vi "Grab images from pco.edge or pco.pixelfly USB with soft ROI.vi"() -> ()   [LabVIEW 2012]
doc: "A short program to demonstrate the fundamentals of control and image acquision with the pco.camera series. The program records a sequence of images, with \"live\" updating, while the \"Record\" button is on. Use ctrl-H for more help on the individual controls and indicators."
panel:
  out "bClose":bool
  in  "Quit":bool
  out "BufNr1":i16
  out "BufNr0":i16
  in  "bUseBuffer1":bool
  in  "bUseBuffer0":bool
  in  "ROIX1":u16=1 min=1
  in  "ROIY1":u16=1 min=1
  in  "ROIY0":u16=1 min=1
  in  "ROIX0":u16=1 min=1
  out "Bits/pixel":u16
  in  "Record":bool
  in  "DelayTimeBase":u16(ring)=2 items=["nanoseconds", "microseconds", "milliseconds"]
  in  "ExposureTimeBase":u16(ring)=2 items=["nanoseconds", "microseconds", "milliseconds"]
  in  "Exposure":u32=10
  in  "Delay":u32
  in  "Rate":i32(ring) items=["12000000", "24000000"]
  out "Image":u16[][](graph)
  in  "TriggerMode":u16(ring) items=["Auto", "Software", "External sequence start ", "External exposure control"]
  # "A short program to demonstrate the fundamentals of control and image acquision with the pco.camera series. The program records a sequence of images, with \"live\" updating, while the \"Record\" button is on.  Use ctrl-H for more help on the individual controls and indicators."
  # "pco.labview"
  # "1) Setup camera:"
  # "2) Record  images:"
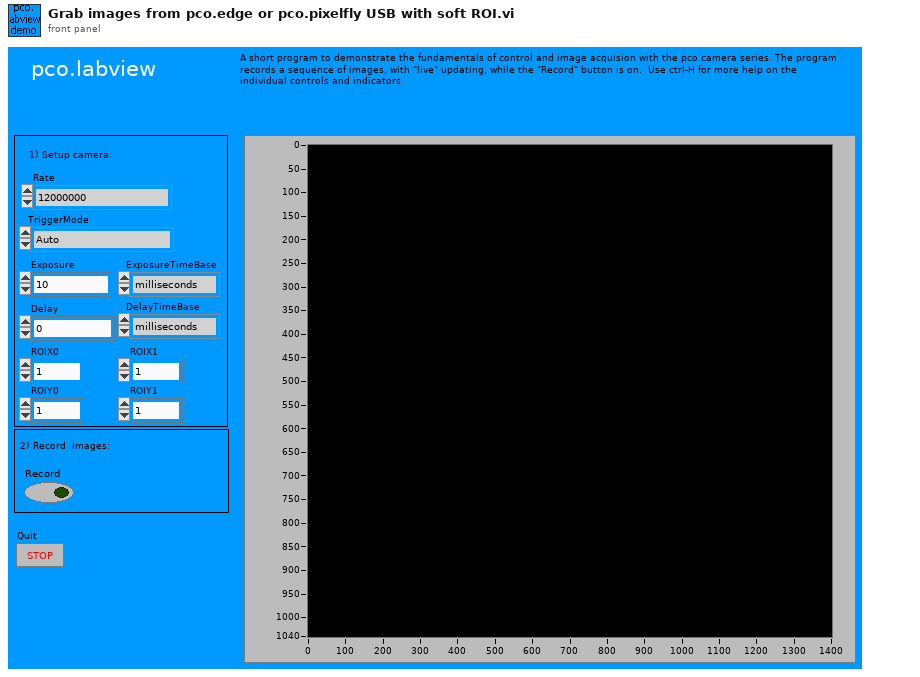
[diagram p1: front panel]
types:
  T1 = cluster{"SSize":u16, "CamType":u16, "CamsSubType":u16, "SerialNumber":u32, "HWVersion":u32, "FWVersion ":u32, "InterfaceType":u16, "HardwareVersions":cluster{"Board":u16, cluster{"string":string, "BatchNumber":u16, "MinorRevision":u8, "MajorRevision":u8, "Variant":u16}[]}, "FirmwareVersions":cluster{"DeviceNum":u16, cluster{"string":string, "MinorRevision":u8, "MajorRevision":u8, "Variant":u16}[]}}
  T2 = cluster{"Size":u16, "SensorTypeDESC":u16, "SensorSubtypeDESC":u16, "MaxHorizontalResStdDESC":u16, "MaxVerticalResStdDESC":u16, "MaxHorizontalResExtDESC":u16, "MaxVerticalResExtDESC":u16, "DynResDESC":u16, "MaxBinHorzDESC":u16, "BinHorzStepDESC":bool, "MaxBinVertDESC":u16, "BinVertStepDESC":bool, "ROIHorzStepDESC":u16, "ROIVertStepDESC":u16, "NumADCDESC":u16, "IRDESC":bool, "MinDelayDESC":u32, "MaxDelayDESC":u32, "MinDelayStepDESC":u32, "MinExpoDESC":u32, "MaxExpoDESC":u32, "MinExpoStepDESC":u32, "MinDelayIRDESC":u32, "MaxDelayIRDESC":u32, "MinExpoIRDESC":u32, "MaxExpoIRDESC":u32, "TimeTableDESC":bool, "DoubleImageDESC":bool, "MinCoolSetDESC":i16, "MaxCoolSetDESC":i16, "MDefaultCoolSetDESC":i16, "PowerDownModeDESC":bool, "OffsetRegDESC":bool, "ColorPattern":cluster{"UpperLeftColor":u8, "UpperRightColor":u8, "LowerLeftColor":u8, "LowerRightColor":u8}, "PatternTypeDESC":bool, "PixelRates":u32[], "CoversionFactors":u16[], "Reserved":u32[], "GeneralCapabilities":u32, "GeneralCapabilities 2":u32, "Min Size Hor":u16, "Min Size Vert":u16, "Ext Synch Freq":u32[], "Cooling Setpoints":i16[], "Soft ROI Hor Step":u16, "Soft ROI Vert Step":u16}
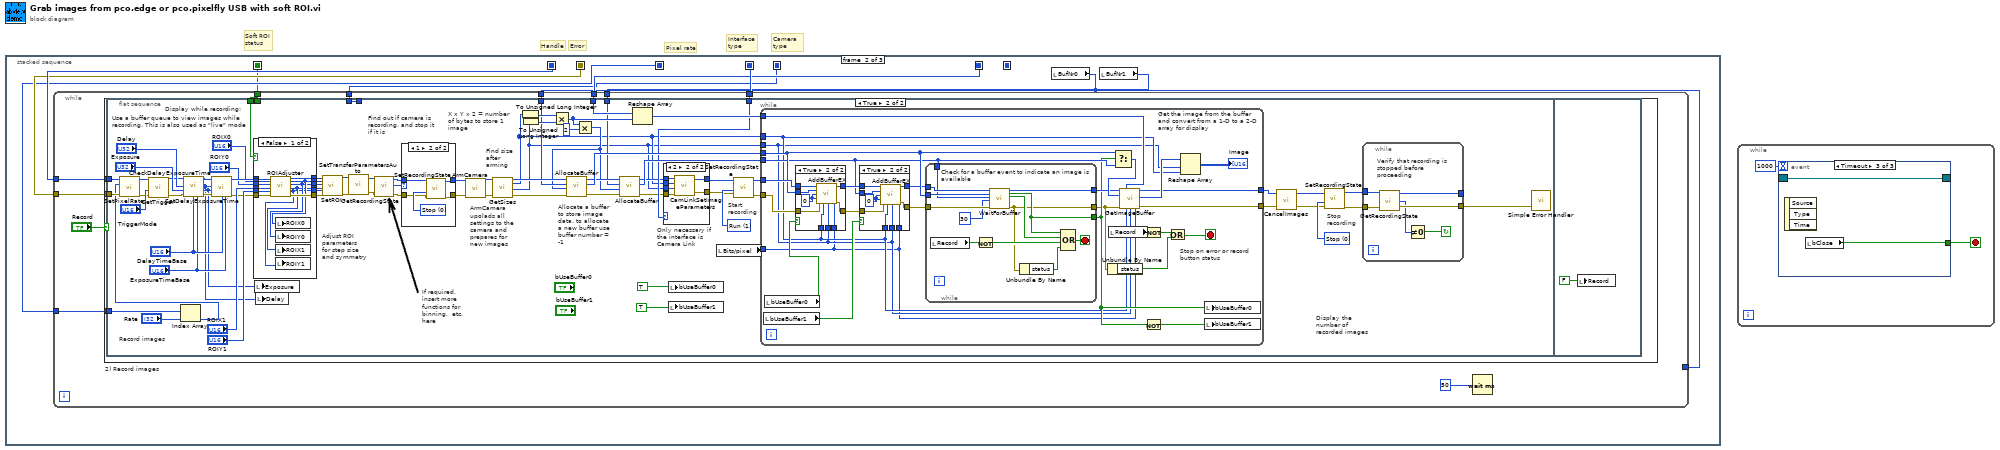
[diagram p0: block diagram]
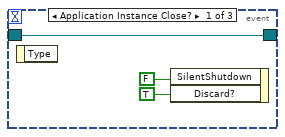
[diagram p2: hidden frame]
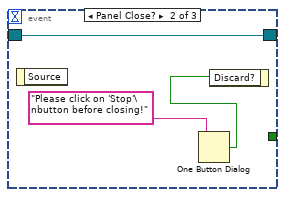
[diagram p3: hidden frame]
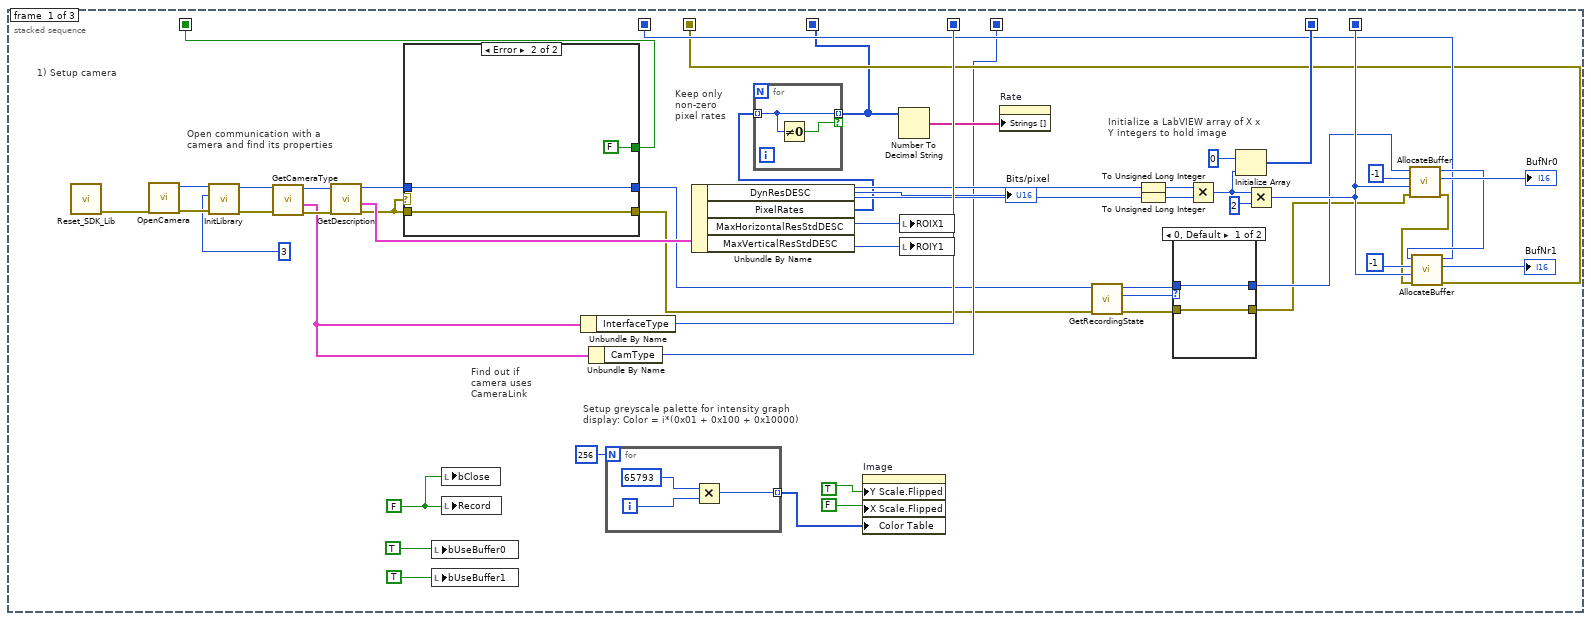
[diagram p4: hidden frame]
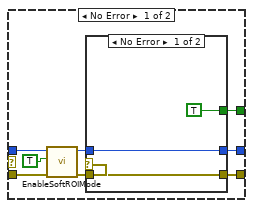
[diagram p5: hidden frame]
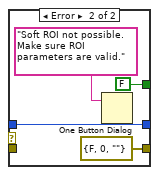
[diagram p6: hidden frame]
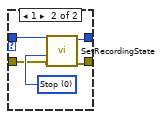
[diagram p7: hidden frame]
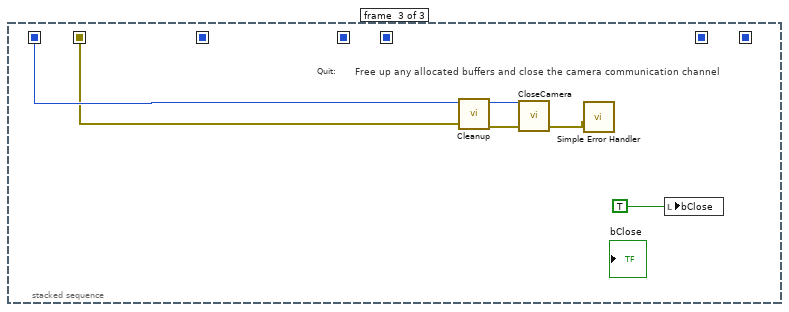
[diagram p14: hidden frame]
diagram:
  # "Soft ROI\nstatus"
  # "Camera type"
  # "Interface type"
  # "Error"
  # "Handle"
  # "Pixel rate"
  n1 = stacked-sequence {
    seq-local: [w44 _ _] -> [_ w86 _]
    seq-local: [w32 _ _] -> [_ _ _]
    seq-local: [w14 _ _] -> [_ w89 w292]
    seq-local: [w13 _ _] -> [_ w88 w291]
    seq-local: [w39 _ _] -> [_ w87 _]
    seq-local: [w1 _ _] -> [_ w83 _]
    seq-local: [w8 _ _] -> [_ w82 _]
    seq-local: [w3 _ _] -> [_ w81 _]
    frame #0 {
      w26 = FALSE ("stop")
      # "Keep only non-zero pixel rates"
      # "1) Setup camera"
      # "Find out if camera uses CameraLink"
      # "Setup greyscale palette for intensity graph display: Color = i*(0x01 + 0x100 + 0x10000)"
      # "Initialize a LabVIEW array of X x Y integers to hold image"
      # "Open communication with a camera and find its properties"
      n2 = call "Reset_SDK_Lib.vi"() -> ("ErrorOut"=w10:errorcluster)  [unwired: 11 in]
      n3 = call "OpenCamera.vi"("ErrorIn"=w10) -> ("ErrorOut"=w23:errorcluster, "Handle out"=w24:u64)  [unwired: 3 in, 2 out]
      n4 = call "InitLibrary.vi"("error in (no error)"=w23, "InterfaceType"=u32 3, "ph"=w24) -> ("error out"=w22:errorcluster, "hout"=w21:u64)  [unwired: 7 in]
      n5 = call "GetCameraType.vi"("ph"=w21, "error in (no error)"=w22) -> ("hout"=w41:u64, "CameraType"=w9:T1, "error out"=w40:errorcluster)  [unwired: 1 in, 1 out]
      n6 = call "GetDescription.vi"("ErrorIn"=w40, "ph"=w41) -> ("ErrorOut"=w4:errorcluster, "Description"=w43:T2, "hout"=w7:u64)  [unwired: 2 in, 1 out]
      n7 = case shown="Error" w4 {
        tunnel: w7 -> [w60 w70]
        tunnel: [w56 w70] -> w6
        tunnel: w4 -> [w58 w69]
        tunnel: [w55 w69] -> w5
        tunnel: [w53 FALSE] -> w3
        frame No Error {
          n8 = call "EnableSoftROIMode.vi"("error in (no error)"=w58, "SoftROI"=TRUE, "ph"=w60) -> ("error out"=w54:errorcluster, "hout"=w57:u64)  [unwired: 3 in, 1 out]
          n9 = case shown="No Error" w54 {
            tunnel: w57 -> [w63 w67]
            tunnel: [w63 w67] -> w56
            tunnel: w54 -> [w62 _]
            tunnel: [w62 errorcluster {"status"=FALSE, "code"=0, "source"=""} ("error out")] -> w55
            tunnel: [TRUE FALSE] -> w53
            frame No Error {
            }
            frame Error {
              n10 = One Button Dialog(message="Soft ROI not possible. Make sure ROI parameters are valid.") -> ()  [unwired: 1 in, 1 out]
            }
          }
        }
        frame Error {
        }
      }
      n11 = local write "bUseBuffer0"(TRUE) -> ()
      n12 = local write "bUseBuffer1"(TRUE) -> ()
      n13 = local write "bClose"(w26) -> ()
      n14 = local write "Record"(w26) -> ()
      n15 = Unbundle By Name(w9) -> ("InterfaceType"=w39:u16)
      n16 = Unbundle By Name(w9) -> ("CamType"=w8:u16)
      n17 = for {
        N: 256 -> [_]
        tunnel: [w78] -> w47 mode=indexing
        i -> [w79]
        n18 = Multiply(x=65793, y=w79) -> (x*y=w78:i32)
      }
      n19 = Unbundle By Name(w43) -> ("DynResDESC"=→"Bits/pixel":u16, "PixelRates"=w2:u32[], "MaxHorizontalResStdDESC"=w37:u16, "MaxVerticalResStdDESC"=w36:u16)
      n20 = for {
        tunnel: w2 -> [w52] mode=indexing
        tunnel: [w52] -> w1 mode=indexing if=w51
        n21 = Not Equal To 0?(x=w52) -> (x != 0?=w51:bool)
      }
      n22 = property on="Image" class="IntGraph (strict)"("Y Scale.Flipped"=TRUE, "X Scale.Flipped"=FALSE, "Color Table"=w47) -> ()  [unwired: 2 in, 2 out]
      n23 = Number To Decimal String(number=w1) -> (decimal integer string=w25:string[])  [unwired: 1 in]
      n24 = local write "ROIX1"(w37) -> ()
      n25 = local write "ROIY1"(w36) -> ()
      n26 = property on="Rate" class="Ring (strict)"("Strings []"=w25) -> ()  [unwired: 2 in, 2 out]
      n27 = call "GetRecordingState.vi"("ErrorIn"=w5, "ph"=w6) -> ("ErrorOut"=w17:errorcluster, "Error"=w11:i32, "hout"=w18:u64)  [unwired: 2 in, 1 out]
      n28 = To Unsigned Long Integer(number=w37) -> (unsigned 32bit integer=w34:u32)
      n29 = To Unsigned Long Integer(number=w36) -> (unsigned 32bit integer=w33:u32)
      n30 = case shown="0, Default" w11 {
        tunnel: w18 -> [w72 w76]
        tunnel: w17 -> [w71 w75]
        tunnel: [w72 w74] -> w16
        tunnel: [w71 w73] -> w12
        frame 0, Default {
        }
        frame 1 {
          w77 = u16 0 items=["Stop", "Run"] ("RecordingState")
          n31 = call "SetRecordingState.vi"("ErrorIn"=w75, "RecordingState"=w77, "ph"=w76) -> ("ErrorOut"=w73:errorcluster, "hout"=w74:u64)  [unwired: 2 in, 1 out]
        }
      }
      n32 = Multiply(x=w34, y=w33) -> (x*y=w45:u32)
      n33 = Initialize Array(u16 0 ("Element Data"), w45) -> (w44:u16[])
      n34 = Multiply(x=w45, y=u32 2) -> (x*y=w32:u32)
      n35 = call "AllocateBuffer.vi"("error in (no error)"=w12, "Size"=w32, "BufNr"=i16 -1, "ph"=w16) -> ("error out"=w19:errorcluster, "BufNrOut"=→"BufNr0":i16, "hout"=w15:u64)  [unwired: 2 in, 3 out]
      n36 = call "AllocateBuffer.vi"("error in (no error)"=w19, "Size"=w32, "BufNr"=i16 -1, "ph"=w15) -> ("error out"=w13:errorcluster, "BufNrOut"=→"BufNr1":i16, "hout"=w14:u64)  [unwired: 2 in, 3 out]
    }
    frame #1 {
      n37 = local read "BufNr0"() -> (w85:i16)
      n38 = local read "BufNr1"() -> (w84:i16)
      n39 = while {
        tunnel: w85 -> [_]
        tunnel: w85 -> [w96]
        tunnel: w86 -> [w98]
        tunnel: w87 -> [w99]
        tunnel: w88 -> [w97]
        tunnel: w89 -> [w94]
        tunnel: w84 -> [w95]
        tunnel: w83 -> [w92]
        tunnel: w82 -> [w91]
        tunnel: w81 -> [w90]
        stop <- "Quit" stop-if-true
        n40 = case "2) Record images" shown="True" "Record" {
          tunnel: w94 -> [_ w110]
          tunnel: w97 -> [_ w109]
          tunnel: w99 -> [_ w103]
          tunnel: w98 -> [_ w108]
          tunnel: w96 -> [_ w107]
          tunnel: w95 -> [_ w106]
          tunnel: w92 -> [_ w105]
          tunnel: w91 -> [_ w104]
          tunnel: w90 -> [_ w102]
          frame False {
          }
          frame True {
            n41 = flat-sequence {
              tunnel: w110 -> [w174]
              tunnel: w109 -> [w173]
              tunnel: w108 -> [w170]
              tunnel: w107 -> [w163]
              tunnel: w106 -> [w159]
              tunnel: w105 -> [w146]
              tunnel: w104 -> [_]
              tunnel: w103 -> [w140]
              tunnel: w102 -> [w121]
              frame #0 {
                w185 = u16 1 items=["Stop", "Run"] ("RecordingState")
                w188 = u16 0 items=["Stop", "Run"] ("RecordingState")
                # "Adjust ROI parameters   for step size and symmetry"
                # "Only necessary if the interface is Camera Link"
                # "Display the number of recorded images"
                # "Record images"
                # "Start recording"
                # "Allocate a buffer to store image data. to allocate a new buffer use buffer number = -1"
                # "Find size after arming"
                # "ArmCamera upolads all settings to the camera and prepares for new images"
                # "Find out if camera is recording, and stop it if it is"
                # "If required, insert more functions for binning.  etc. here"
                # "X x Y x 2 = number of bytes to store 1 image"
                # "Stop recording"
                # "Use a buffer queue to view images while recording. This is also used as \"live\" mode"
                # "Display while recording:"
                n42 = Index Array(array=w146, index="Rate") -> (element=w145:u32)
                n43 = call "SetPixelRate.vi"("error in (no error)"=w173, "PixelRate"=w145, "ph"=w174) -> ("error out"=w148:errorcluster, "hout"=w149:u64)  [unwired: 2 in, 1 out]
                n44 = call "SetTrigger.vi"("error in (no error)"=w148, "TriggerMode"="TriggerMode", "ph"=w149) -> ("error out"=w117:errorcluster, "hout"=w118:u64)  [unwired: 2 in, 1 out]
                n45 = call "CheckDelayExposureTime.vi"("ph"=w118, "Delay"="Delay", "Exposure"="Exposure", "error in (no error)"=w117, "DelayTimeBase"="DelayTimeBase", "ExposureTimeBase"="ExposureTimeBase") -> ("hout"=w115:u64, "Delay Out"=w111:u32, "Exposure Out"=w112:u32, "error out"=w116:errorcluster)  [unwired: 4 in, 2 out]
                n46 = call "SetDelayExposureTime.vi"("ph"=w115, "Delay"=w111, "Exposure"=w112, "error in (no error)"=w116, "DelayTimeBase"="DelayTimeBase", "ExposureTimeBase"="ExposureTimeBase") -> ("hout"=w133:u64, "error out"=w123:errorcluster)  [unwired: 7 in, 1 out]
                n47 = case shown="False" w121 {
                  tunnel: w133 -> [w200 w206]
                  tunnel: [w199 w206] -> w132
                  tunnel: "ROIX0" -> [w198 w205]
                  tunnel: "ROIY0" -> [w197 w204]
                  tunnel: "ROIX1" -> [w196 w203]
                  tunnel: "ROIY1" -> [w195 w202]
                  tunnel: [w192 w205] -> w127
                  tunnel: [w191 w204] -> w126
                  tunnel: [w190 w203] -> w125
                  tunnel: [w189 w202] -> w124
                  tunnel: w123 -> [w194 w201]
                  tunnel: [w193 w201] -> w122
                  frame False {
                    n48 = call "ROIAdjuster.vi"("HandleIn"=w200, "ROIXmin"=w198, "ROIYmin"=w197, "ROIXmax"=w196, "ROIYmax"=w195, "ErrorIn"=w194) -> ("hout"=w199:u64, "ROIX0Mod"=w192:u16, "ROIY0Mod"=w191:u16, "ROIX1Mod"=w190:u16, "ROIY1Mod"=w189:u16, "ErrorOut"=w193:errorcluster)  [unwired: 7 in, 1 out]
                    n49 = local write "ROIX0"(w192) -> ()
                    n50 = local write "ROIY0"(w191) -> ()
                    n51 = local write "ROIX1"(w190) -> ()
                    n52 = local write "ROIY1"(w189) -> ()
                  }
                  frame True {
                  }
                }
                n53 = local write "Exposure"(w112) -> ()
                n54 = local write "Delay"(w111) -> ()
                n55 = call "SetROI.vi"("ph"=w132, "ROIX0"=w127, "ROIY0"=w126, "ROIX1"=w125, "ROIY1"=w124, "error in (no error)"=w122) -> ("hout"=w144:u64, "error out"=w143:errorcluster)  [unwired: 12 in]
                n56 = call "SetTransferParametersAuto.vi"("error in (no error)"=w143, "ph"=w144) -> ("error out"=w142:errorcluster, "hout"=w141:u64)  [unwired: 2 in, 1 out]
                n57 = call "GetRecordingState.vi"("ErrorIn"=w142, "ph"=w141) -> ("ErrorOut"=w182:errorcluster, "RecordingState"=w184:u16, "hout"=w183:u64)  [unwired: 2 in, 1 out]
                n58 = case shown="1" w184 {
                  tunnel: w183 -> [w284 w288]
                  tunnel: w182 -> [w283 w287]
                  tunnel: [w284 w286] -> w181
                  tunnel: [w283 w285] -> w180
                  frame 0, Default {
                  }
                  frame 1 {
                    w289 = u16 0 items=["Stop", "Run"] ("RecordingState")
                    n59 = call "SetRecordingState.vi"("ErrorIn"=w287, "RecordingState"=w289, "ph"=w288) -> ("ErrorOut"=w285:errorcluster, "hout"=w286:u64)  [unwired: 2 in, 1 out]
                  }
                }
                n60 = call "ArmCamera.vi"("error in (no error)"=w180, "ph"=w181) -> ("error out"=w178:errorcluster, "hout"=w179:u64)  [unwired: 1 in, 1 out]
                n61 = call "GetSizes.vi"("ph"=w179, "ErrorIn"=w178) -> ("hout"=w175:u64, "XResAct"=w135:u16, "YResAct"=w134:u16, "ErrorOut"=w177:errorcluster)  [unwired: 11 in, 3 out]
                n62 = To Unsigned Long Integer(number=w135) -> (unsigned 32bit integer=w164:u32)
                n63 = To Unsigned Long Integer(number=w134) -> (unsigned 32bit integer=w165:u32)
                n64 = Multiply(x=w164, y=w165) -> (x*y=w166:u32)
                n65 = Multiply(x=w166, y=u32 2) -> (x*y=w160:u32)
                n66 = call "AllocateBuffer.vi"("error in (no error)"=w177, "Size"=w160, "BufNr"=w163, "ph"=w175) -> ("error out"=w162:errorcluster, "BufNrOut"=w167:i16, "hout"=w161:u64)  [unwired: 2 in, 3 out]
                n67 = call "AllocateBuffer.vi"("error in (no error)"=w162, "Size"=w160, "BufNr"=w159, "ph"=w161) -> ("error out"=w137:errorcluster, "BufNrOut"=w158:i16, "hout"=w139:u64)  [unwired: 2 in, 3 out]
                n68 = Reshape Array(w170, w166) -> (w169:u16[])
                n69 = case shown="2" w140 {
                  tunnel: w139 -> [w208 w214]
                  tunnel: [w208 w213] -> w138
                  tunnel: w137 -> [w207 w212]
                  tunnel: [w207 w211] -> w136
                  tunnel: w135 -> [_ w210]
                  tunnel: w134 -> [_ w209]
                  frame 0, Default {
                  }
                  frame 2 {
                    n70 = call "CamLinkSetImageParameters.vi"("error in (no error)"=w212, "YRes"=w209, "XRes"=w210, "ph"=w214) -> ("error out"=w211:errorcluster, "hout"=w213:u64)  [unwired: 1 out]
                  }
                }
                n71 = local write "bUseBuffer0"(TRUE) -> ()
                n72 = local write "bUseBuffer1"(TRUE) -> ()
                n73 = local read "Bits/pixel"() -> (w153:u16)
                n74 = call "SetRecordingState.vi"("ErrorIn"=w136, "RecordingState"=w185, "ph"=w138) -> ("ErrorOut"=w172:errorcluster, "hout"=w171:u64)  [unwired: 2 in, 1 out]
                n75 = while {
                  tunnel: w167 -> [w227]
                  tunnel: w169 -> [w237]
                  tunnel: w171 -> [w236]
                  tunnel: w134 -> [w216]
                  tunnel: w135 -> [w217]
                  tunnel: w172 -> [w234]
                  tunnel: [w239] -> w152
                  tunnel: [w240] -> w151
                  tunnel: w158 -> [w226]
                  tunnel: w153 -> [w215]
                  stop <- w218 stop-if-true
                  # "Stop on error or record button status"
                  # "Get the image from the buffer and convert from a 1-D to a 2-D array for display"
                  n76 = local read "bUseBuffer1"() -> (w231:bool)
                  n77 = local read "bUseBuffer0"() -> (w232:bool)
                  n78 = case shown="True" w232 {
                    tunnel: [w243 w252] -> w233
                    tunnel: [w242 w251] -> w235
                    tunnel: w227 -> [_ w250]
                    tunnel: w236 -> [w242 w249]
                    tunnel: w215 -> [_ w247]
                    tunnel: w217 -> [_ w246]
                    tunnel: w216 -> [_ w245]
                    tunnel: w234 -> [w243 w244]
                    frame False {
                    }
                    frame True {
                      w248 = i16 0
                      n79 = call "AddBufferEX.vi"("ph"=w249, "BuffNr"=w250, "1stImage"=w248, "LastImage"=w248, "error in (no error)"=w244, "XRes"=w246, "YRes"=w245, "BitPerPixel"=w247) -> ("hout"=w251:u64, "error out"=w252:errorcluster)  [unwired: 5 in, 1 out]
                    }
                  }
                  n80 = case shown="True" w231 {
                    tunnel: [w253 w263] -> w224
                    tunnel: [w254 w262] -> w225
                    tunnel: w226 -> [_ w261]
                    tunnel: w235 -> [w254 w260]
                    tunnel: w215 -> [_ w258]
                    tunnel: w217 -> [_ w257]
                    tunnel: w216 -> [_ w256]
                    tunnel: w233 -> [w253 w255]
                    frame False {
                    }
                    frame True {
                      w259 = i16 0
                      n81 = call "AddBufferEX.vi"("ph"=w260, "BuffNr"=w261, "1stImage"=w259, "LastImage"=w259, "error in (no error)"=w255, "XRes"=w257, "YRes"=w256, "BitPerPixel"=w258) -> ("hout"=w262:u64, "error out"=w263:errorcluster)  [unwired: 5 in, 1 out]
                    }
                  }
                  n82 = while {
                    tunnel: w227 -> [w271]
                    tunnel: w226 -> [w270]
                    tunnel: w225 -> [w273]
                    tunnel: w224 -> [w272]
                    tunnel: [w269] -> w223
                    tunnel: [w265] -> w221
                    tunnel: [w268] -> w222
                    stop <- w274 stop-if-true
                    # "Check for a buffer event to indicate an image is available"
                    n83 = local read "Record"() -> (w276:bool)
                    n84 = Not(x=w276) -> (.not. x?=w275:bool)
                    n85 = call "WaitForBuffer.vi"("ph"=w273, "sBufNr"=w271, "sBufNr 2"=w270, "timeout"=30, "error in (no error)"=w272) -> ("hout"=w269:u64, "Buffer_Ready"=w268:bool, "Buffer_Ready 2"=w267:bool, "error out"=w265:errorcluster)  [unwired: 10 in, 1 out]
                    n86 = Unbundle By Name(w265) -> ("status"=w264:bool)
                    n87 = Compound Arithmetic op=OR(w268, w267, w275, w264) -> (w274:bool)
                  }
                  n88 = Unbundle By Name(w221) -> ("status"=w219:bool)
                  n89 = local read "Record"() -> (w238:bool)
                  n90 = Select(t=w227, s=w222, f=w226) -> (s? t:f=w230:i16)
                  n91 = call "GetImageBuffer.vi"("ph"=w223, "BuffIn"=w237, "BuffNr"=w230, "error in (no error)"=w221, "xRes"=w217, "yRes"=w216, "Bitresolution"=w215) -> ("hout"=w239:u64, "BuffOut"=w241:u16[], "error out"=w240:errorcluster)  [unwired: 5 in, 1 out]
                  n92 = Not(x=w222) -> (.not. x?=w229:bool)
                  n93 = Not(x=w238) -> (.not. x?=w220:bool)
                  n94 = Or(x=w220, y=w219) -> (x .or. y?=w218:bool)
                  n95 = Reshape Array(w241, w216, w217) -> (→"Image":u16[][])
                  n96 = local write "bUseBuffer0"(w222) -> ()
                  n97 = local write "bUseBuffer1"(w229) -> ()
                }
                n98 = call "CancelImages.vi"("error in (no error)"=w151, "ph"=w152) -> ("error out"=w155:errorcluster, "hout"=w154:u64)  [unwired: 1 in, 1 out]
                n99 = call "SetRecordingState.vi"("ErrorIn"=w155, "RecordingState"=w188, "ph"=w154) -> ("ErrorOut"=w186:errorcluster, "hout"=w187:u64)  [unwired: 2 in, 1 out]
                n100 = while {
                  tunnel: [w280] -> w150
                  tunnel: w186 -> [w281]
                  tunnel: w187 -> [w282]
                  tunnel: [w277] -> _
                  stop <- w278 continue-if-true
                  # "Verify that recording is stopped before proceeding"
                  n101 = call "GetRecordingState.vi"("ErrorIn"=w281, "ph"=w282) -> ("ErrorOut"=w280:errorcluster, "RecordingState"=w279:u16, "hout"=w277:u64)  [unwired: 2 in, 1 out]
                  n102 = Not Equal To 0?(x=w279) -> (x != 0?=w278:bool)
                }
                n103 = call <vilib>:"Simple Error Handler.vi"("error in (no error)"=w150) -> ()  [unwired: 4 in, 5 out]
              }
              frame #1 {
                n104 = local write "Record"(FALSE ("Record")) -> ()
              }
            }
          }
        }
        n105 = Wait (ms)(milliseconds to wait=u32 50) -> ()  [unwired: 1 out]
      }
    }
    frame #2 {
      # "Free up any allocated buffers and close the camera communication channel"
      # "Quit:"
      n106 = call "Cleanup.vi"("error in (no error)"=w291, "ph"=w292) -> ("error out"=w293:errorcluster, "hout"=w294:u64)  [unwired: 8 in]
      n107 = call "CloseCamera.vi"("ErrorIn"=w293, "Handle in"=w294) -> ("ErrorOut"=w296:errorcluster)  [unwired: 1 in, 2 out]
      n108 = call <vilib>:"Simple Error Handler.vi"("error in (no error)"=w296) -> ()  [unwired: 4 in, 5 out]
      n109 = local write "bClose"(TRUE) -> ()
    }
  }
  n110 = while {
    stop <- w297 stop-if-true
    n111 = event shown="[2] Timeout" {
      selector: _ -> [w299 w304 w306]
      dyn-events: [w299 w304 w306] -> _
      timeout: 1000 -> [_ _ _]
      tunnel: [_ _ w305] -> w297
      event Application Instance Close? {
        n112 = event-data() -> ()  [unwired: 1 in, 1 out]
        n113 = event-data("SilentShutdown"=FALSE, "Discard?"=TRUE) -> ()  [unwired: 1 in, 1 out]
      }
      event Panel Close? {
        n114 = event-data() -> ()  [unwired: 1 in, 1 out]
        n115 = One Button Dialog(message="Please click on 'Stop'\nbutton before closing!") -> (true=w302:bool)  [unwired: 1 in]
        n116 = event-data("Discard?"=w302) -> ()  [unwired: 1 in, 1 out]
      }
      event Timeout {
        n117 = event-data() -> ()  [unwired: 1 in, 3 out]
        n118 = local read "bClose"() -> (w305:bool)
      }
    }
  }
